vi "Read NewOff1.lvclass.vi"(8 "error in (no error)":errorcluster, 11 "Playbook in":refnum<class "Playbook.lvclass">) -> (0 "error out":errorcluster, 2 "NewOff1.lvclass":refnum<class "NewOff1.lvclass">, 3 "Playbook out":refnum<class "Playbook.lvclass">)   [LabVIEW 2022 SP3]
uses:
  Playbook.lvclass
  NewOff1/NewOff1.lvclass
  C:/Users/ebert/Documents/codes/SSL/repo/SSL_AI/Play_class/Play.lvclass
  C:/Users/ebert/Documents/codes/SSL/repo/SSL_AI/NewOff1/NewOff1.lvclass
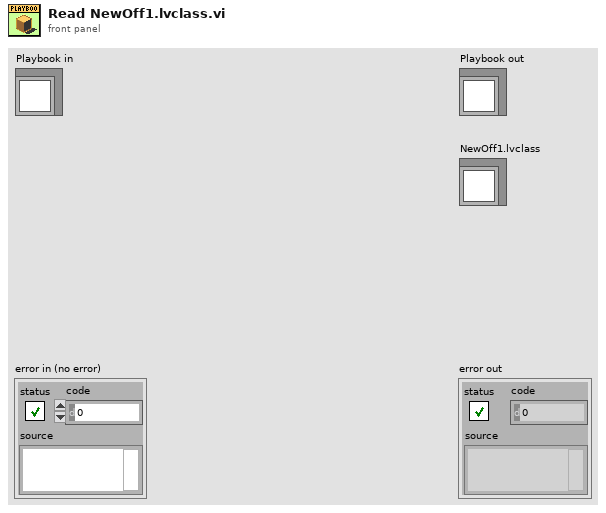
[diagram p1: front panel]
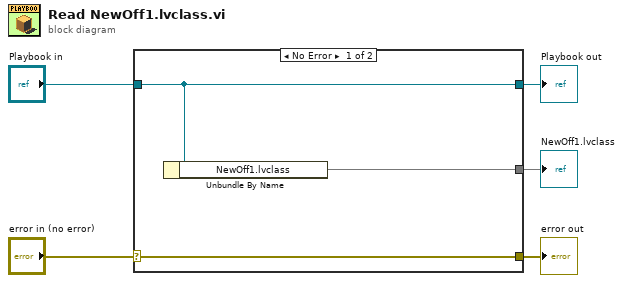
[diagram p0: block diagram]
diagram:
  n1 = case shown="No Error" "error in (no error)" {
    selector: "error in (no error)" -> [w8 w9]
    tunnel: [w8 w9] -> w4
    tunnel: [w7 w10] -> w2
    tunnel: "Playbook in" -> [w7 w10]
    tunnel: [w6 _] -> w1
    frame No Error {
      n2 = Unbundle By Name(w7) -> ("NewOff1.lvclass"=w6)
    }
    frame Error {
    }
  }
  "error out" <- w4
  "Playbook out" <- w2
  "NewOff1.lvclass" <- w1
